vi "Build URI String.vi"(4 "URI Components":T1, 5 "Query Map":map{string, string}(c390)) -> (7 "URI String":string)   [LabVIEW 2020, in "URI.lvlib"]
uses:
  URI.lvlib
  URI Components.ctl
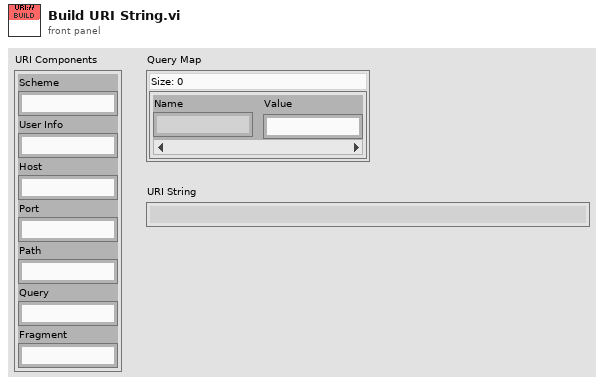
[diagram p1: front panel]
types:
  T1 = typedef "URI.lvlib/URI Components.ctl" = cluster{"Scheme":string, "User Info":string, "Host":string, "Port":string, "Path":string, "Query":string, "Fragment":string}
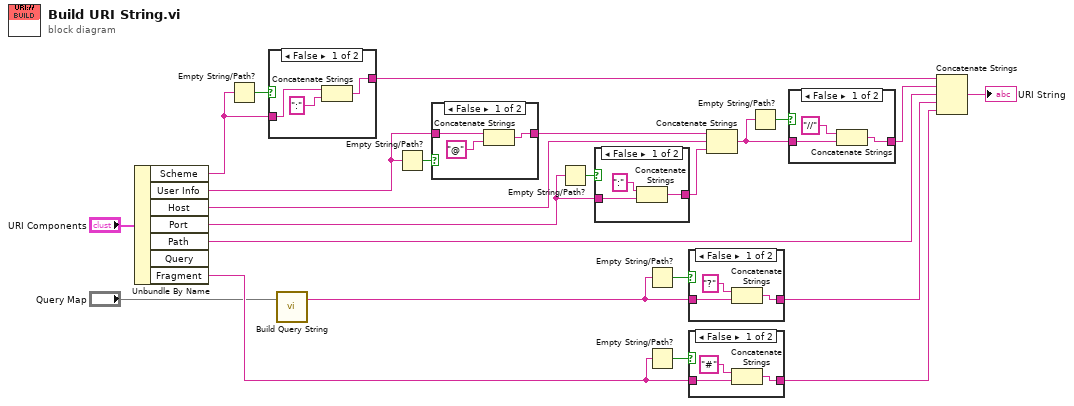
[diagram p0: block diagram]
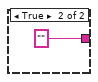
[diagram p6: hidden frame]
diagram:
  n1 = Unbundle By Name("URI Components") -> ("Scheme"=w22:string, "User Info"=w5:string, "Host"=w18:string, "Port"=w20:string, "Path"=w13:string, "Fragment"=w9:string)  [unwired: 1 out]
  n2 = Empty String/Path?(string/path=w22) -> (empty?=w23:bool)
  n3 = case shown="False" w23 {
    tunnel: w22 -> [w26 _]
    tunnel: [w24 ""] -> w15
    frame False {
      n4 = Concatenate Strings(w26, ":" ("string")) -> (w24:string)
    }
    frame True {
    }
  }
  n5 = call "Build Query String.vi"("Query Map"="Query Map") -> ("Query String"=w1:string)  [unwired: 6 in]
  n6 = Empty String/Path?(string/path=w5) -> (empty?=w6:bool)
  n7 = case shown="False" w6 {
    tunnel: w5 -> [w30 w31]
    tunnel: [w28 w31] -> w7
    frame False {
      n8 = Concatenate Strings(w30, "@" ("string")) -> (w28:string)
    }
    frame True {
    }
  }
  n9 = Empty String/Path?(string/path=w20) -> (empty?=w21:bool)
  n10 = case shown="False" w21 {
    tunnel: w20 -> [w34 w35]
    tunnel: [w32 w35] -> w19
    frame False {
      n11 = Concatenate Strings(":" ("string"), w34) -> (w32:string)
    }
    frame True {
    }
  }
  n12 = Empty String/Path?(string/path=w1) -> (empty?=w12:bool)
  n13 = Empty String/Path?(string/path=w9) -> (empty?=w10:bool)
  n14 = case shown="False" w12 {
    tunnel: w1 -> [w38 w39]
    tunnel: [w36 w39] -> w11
    frame False {
      n15 = Concatenate Strings("?" ("string"), w38) -> (w36:string)
    }
    frame True {
    }
  }
  n16 = case shown="False" w10 {
    tunnel: w9 -> [w42 w43]
    tunnel: [w40 w43] -> w8
    frame False {
      n17 = Concatenate Strings("#" ("string"), w42) -> (w40:string)
    }
    frame True {
    }
  }
  n18 = Concatenate Strings(w7, w18, w19) -> (w16:string)
  n19 = Empty String/Path?(string/path=w16) -> (empty?=w17:bool)
  n20 = case shown="False" w17 {
    tunnel: w16 -> [w46 w47]
    tunnel: [w44 w47] -> w14
    frame False {
      n21 = Concatenate Strings("//" ("string"), w46) -> (w44:string)
    }
    frame True {
    }
  }
  n22 = Concatenate Strings(w15, w14, w13, w11, w8) -> (→"URI String":string)
